vi "Hadamard vs DAQ (1).vi"() -> ()   [LabVIEW 2023]
uses:
  <vilib>/Utility/miscctls.llb/LVBoundsTypeDef.ctl
  <vilib>/Utility/miscctls.llb/LVRectTypeDef.ctl
panel:
  in  "Plot Area:Size":T1
  out "?":errorcluster
  in  "error in (no error)":errorcluster
  in  "Z Scale.Marker Values[]":cluster{dbl, u32}[](array[cluster])=[{0.0, 0}, {100.0, 16777215}]
  out "Delay":i32=20
  out "Intensity Graph":dbl[][](graph)=[[0.0, 1.0, 0.0, 1.0, 1.0, 0.0, 1.0, 0.0, 0.0, 1.0, 0.0, 1.0, 1.0, 0.0, 1.0, 0.0], [0.0, 1.0, 0.0, 1.0, 1.0, 0.0, 1.0, 0.0, 0.0, 1.0, 0.0, 1.0, 1.0, 0.0, 1.0, 0.0], [1.0, 0.0, 1.0, 0.0, 0.0, 1.0, 0.0, 1.0, 1.0, 0.0, 1.0, 0.0, 0.0, 1.0, 0.0, 1.0], [1.0, 0.0, 1.0, 0.0, 0.0, 1.0, 0.0, 1.0, 1.0, 0.0, 1.0, 0.0, 0.0, 1.0, 0.0, 1.0], [0.0, 1.0, 0.0, 1.0, 1.0, 0.0, 1.0, 0.0, 0.0, 1.0, 0.0, 1.0, 1.0, 0.0, 1.0, 0.0], [0.0, 1.0, 0.0, 1.0, 1.0, 0.0, 1.0, 0.0, 0.0, 1.0, 0.0, 1.0, 1.0, 0.0, 1.0, 0.0], [1.0, 0.0, 1.0, 0.0, 0.0, 1.0, 0.0, 1.0, 1.0, 0.0, 1.0, 0.0, 0.0, 1.0, 0.0, 1.0], [1.0, 0.0, 1.0, 0.0, 0.0, 1.0, 0.0, 1.0, 1.0, 0.0, 1.0, 0.0, 0.0, 1.0, 0.0, 1.0], [0.0, 1.0, 0.0, 1.0, 1.0, 0.0, 1.0, 0.0, 0.0, 1.0, 0.0, 1.0, 1.0, 0.0, 1.0, 0.0], [0.0, 1.0, 0.0, 1.0, 1.0, 0.0, 1.0, 0.0, 0.0, 1.0, 0.0, 1.0, 1.0, 0.0, 1.0, 0.0], [1.0, 0.0, 1.0, 0.0, 0.0, 1.0, 0.0, 1.0, 1.0, 0.0, 1.0, 0.0, 0.0, 1.0, 0.0, 1.0], [1.0, 0.0, 1.0, 0.0, 0.0, 1.0, 0.0, 1.0, 1.0, 0.0, 1.0, 0.0, 0.0, 1.0, 0.0, 1.0], [0.0, 1.0, 0.0, 1.0, 1.0, 0.0, 1.0, 0.0, 0.0, 1.0, 0.0, 1.0, 1.0, 0.0, 1.0, 0.0], [0.0, 1.0, 0.0, 1.0, 1.0, 0.0, 1.0, 0.0, 0.0, 1.0, 0.0, 1.0, 1.0, 0.0, 1.0, 0.0], [1.0, 0.0, 1.0, 0.0, 0.0, 1.0, 0.0, 1.0, 1.0, 0.0, 1.0, 0.0, 0.0, 1.0, 0.0, 1.0], [1.0, 0.0, 1.0, 0.0, 0.0, 1.0, 0.0, 1.0, 1.0, 0.0, 1.0, 0.0, 0.0, 1.0, 0.0, 1.0]]
  out "N":i32=16
  in  "stop":bool
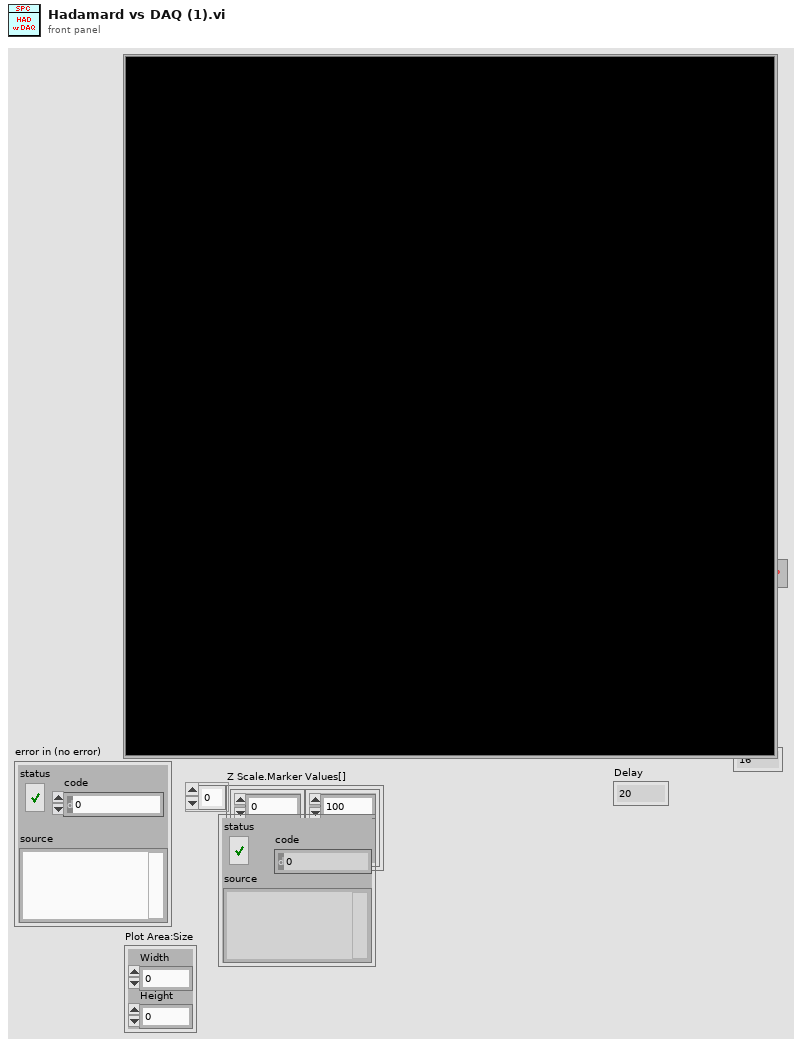
[diagram p1: front panel]
types:
  T1 = typedef "LVBoundsTypeDef.ctl" = cluster{"Width":u32, "Height":u32}
  T2 = typedef "LVRectTypeDef.ctl" = cluster{"Left":i16, "Top":i16, "Right":i16, "Bottom":i16}
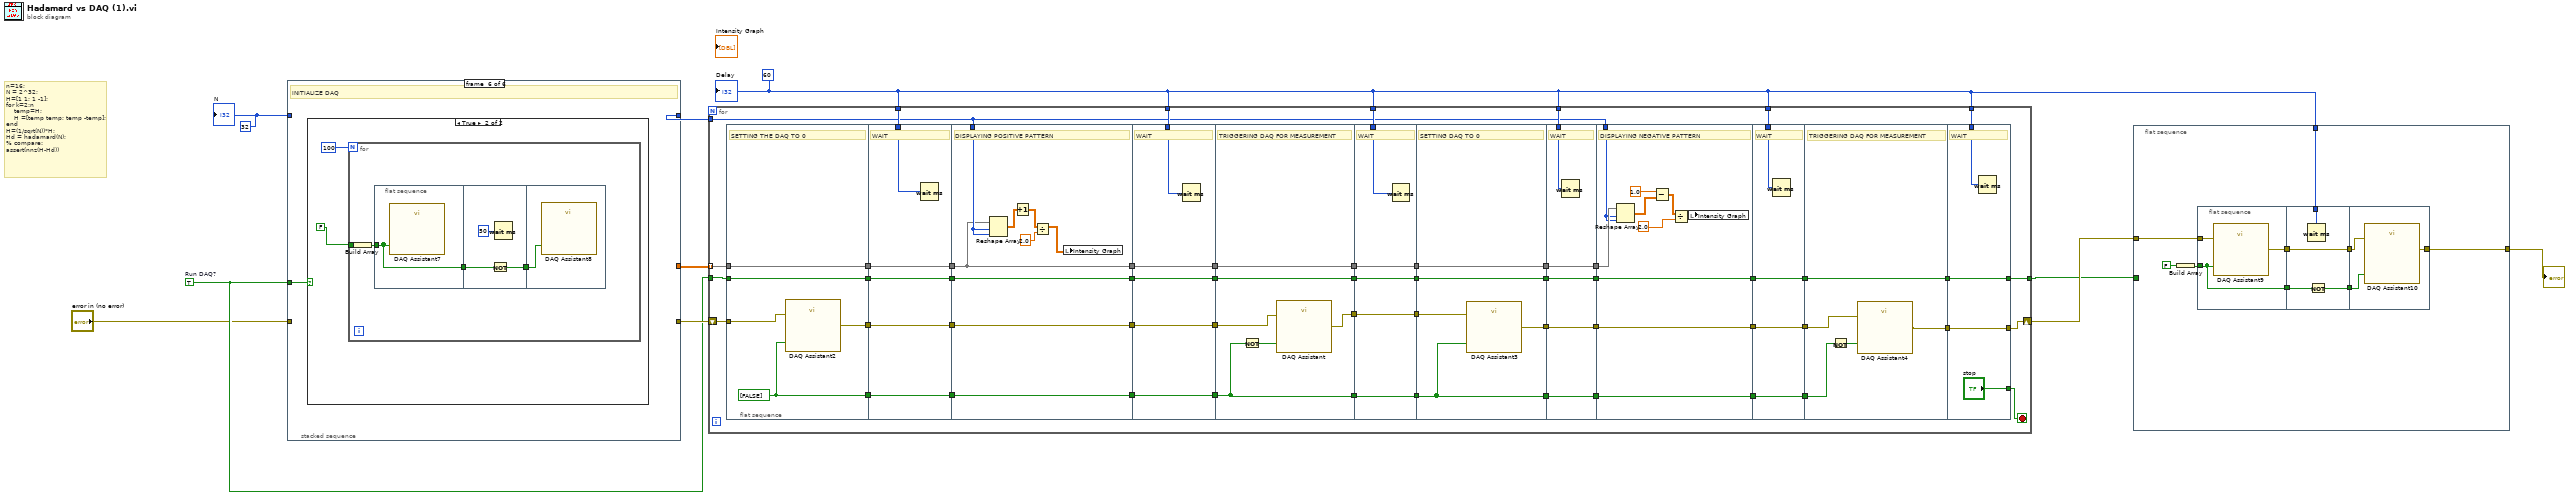
[diagram p0: block diagram]
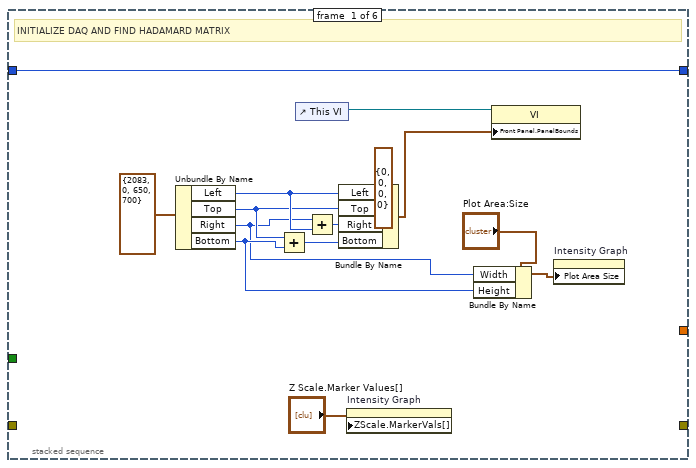
[diagram p2: hidden frame]
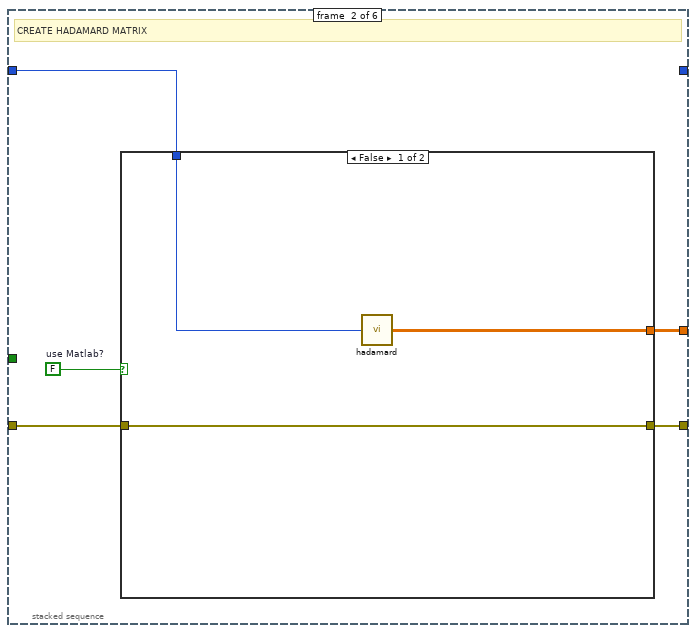
[diagram p3: hidden frame]
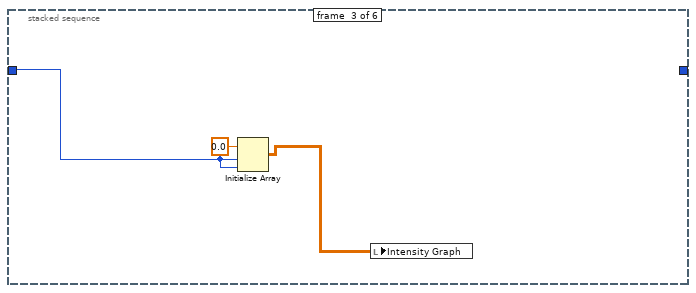
[diagram p5: hidden frame]
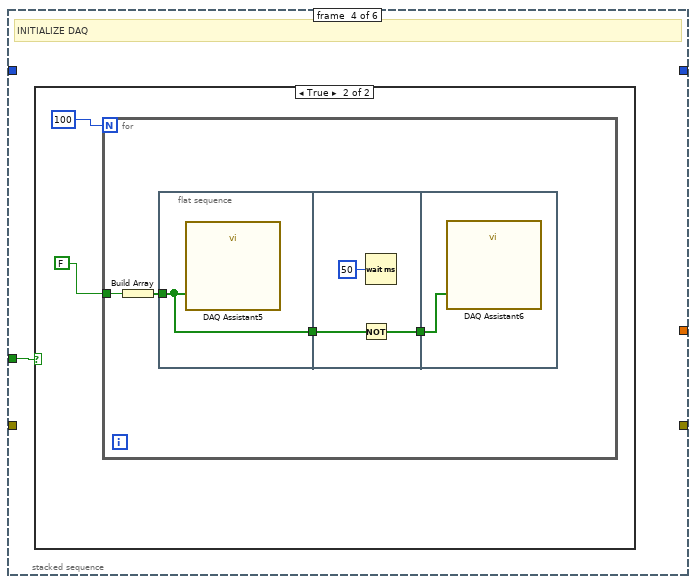
[diagram p6: hidden frame]
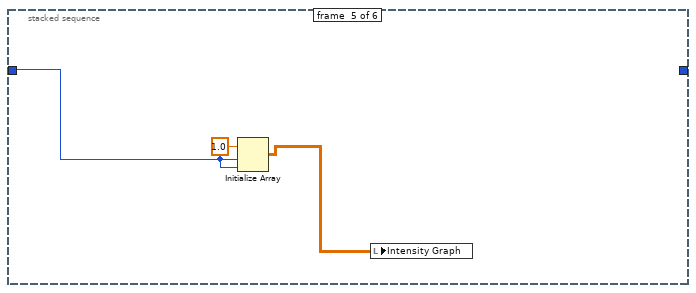
[diagram p8: hidden frame]
diagram:
  w4 = TRUE  # Run DAQ?
  w3 = 60 ("Delay")
  w7 = 32 ("N")
  # "n=16;\nN = 2^32;\nH=[1 1; 1 -1];\nfor k=2:n\n    temp=H;\n    H =[temp temp; temp -temp];\nend\nH=(1/sqrt(N))*H;\nHd = hadamard(N);\n% compare:\nassert(nnz(H-Hd))"
  n1 = stacked-sequence {
    tunnel: [_ w25 _ _ _ _] -> w9
    tunnel: w7 -> [w24 w28 w36 _ w51 _]
    tunnel: [w24 _ _ _ _ _] -> w8
    tunnel: [_ w27 _ _ _ _] -> w10
    tunnel: w4 -> [_ _ _ w37 _ w52]
    tunnel: "error in (no error)" -> [_ w26 _ _ _ _]
    frame #0 {
      # "INITIALIZE DAQ AND FIND HADAMARD MATRIX"
      n2 = Unbundle By Name(T2 {"Left"=2083, "Top"=0, "Right"=650, "Bottom"=700} ("Front Panel Window:Panel Bounds")) -> ("Left"=w20:i16, "Top"=w12:i16, "Right"=w11:i16, "Bottom"=w13:i16)
      n3 = Add(x=w12, y=w13) -> (x+y=w17:i16)
      n4 = control-ref of="This VI"() -> (w22:refnum<vi>)
      n5 = Add(x=w11, y=w20) -> (x+y=w19:i16)
      n6 = Bundle By Name(cluster=T2 {"Left"=0, "Top"=0, "Right"=0, "Bottom"=0} ("output cluster"), "Left"=w20, "Top"=w12, "Right"=w19, "Bottom"=w17) -> (w18:T2)
      n7 = property on="Intensity Graph" class="IntGraph (strict)"("ZScale.MarkerVals[]"="Z Scale.Marker Values[]") -> ()  [unwired: 2 in, 2 out]
      n8 = Bundle By Name(cluster="Plot Area:Size", "Width"=w11, "Height"=w13) -> (w14:T1)
      n9 = property class="VI"(reference=w22, "Front Panel.PanelBounds"=w18) -> ()  [unwired: 1 in, 2 out]
      n10 = property on="Intensity Graph" class="IntGraph (strict)"("Plot Area Size"=w14) -> ()  [unwired: 2 in, 2 out]
    }
    frame #1 {
      w29 = FALSE  # use Matlab?
      # "CREATE HADAMARD MATRIX"
      n11 = case shown="False" w29 {
        tunnel: w28 -> [w32 _]
        tunnel: [w31 _] -> w25
        tunnel: [w30 w33] -> w27
        tunnel: w26 -> [w30 w33]
        frame False {
          n12 = call "hadamard.vi"("N"=w32) -> ("Intensity Graph"=w31:dbl[][])
        }
        frame True {
          # "Copy this code to the matlab window"
        }
      }
    }
    frame #2 {
      n13 = Initialize Array(0.0 ("element"), w36, w36) -> (w35:dbl[][])
      n14 = local write "Intensity Graph"(w35) -> ()
    }
    frame #3 {
      # "INITIALIZE DAQ"
      n15 = case shown="True" w37 {
        frame False {
        }
        frame True {
          n16 = for {
            N: 100 -> [_]
            tunnel: FALSE -> [w42]
            n17 = Build Array(w42) -> (w43:bool[])
            n18 = flat-sequence {
              tunnel: w43 -> [w44]
              tunnel: [w44] -> w40
              tunnel: [w45] -> w41
              tunnel: w40 -> [w46]
              tunnel: w41 -> [w48]
              frame #0 {
                n19 = call "DAQ Assistant5"("data"=w44) -> ()  [unwired: 17 in, 2 out]
              }
              frame #1 {
                n20 = Not(x=w46) -> (.not. x?=w45:bool[])
                n21 = Wait (ms)(milliseconds to wait=u32 50) -> ()  [unwired: 1 out]
              }
              frame #2 {
                n22 = call "DAQ Assistant6"("data"=w48) -> ()  [unwired: 17 in, 2 out]
              }
            }
          }
        }
      }
    }
    frame #4 {
      n23 = Initialize Array(1.0 ("element"), w51, w51) -> (w50:dbl[][])
      n24 = local write "Intensity Graph"(w50) -> ()
    }
    frame #5 {
      # "INITIALIZE DAQ"
      n25 = case shown="True" w52 {
        frame False {
        }
        frame True {
          n26 = for {
            N: 100 -> [_]
            tunnel: FALSE -> [w57]
            n27 = Build Array(w57) -> (w58:bool[])
            n28 = flat-sequence {
              tunnel: w58 -> [w59]
              tunnel: [w59] -> w55
              tunnel: [w60] -> w56
              tunnel: w55 -> [w61]
              tunnel: w56 -> [w63]
              frame #0 {
                n29 = call "DAQ Assistant7"("data"=w59) -> ()  [unwired: 17 in, 2 out]
              }
              frame #1 {
                n30 = Not(x=w61) -> (.not. x?=w60:bool[])
                n31 = Wait (ms)(milliseconds to wait=u32 50) -> ()  [unwired: 1 out]
              }
              frame #2 {
                n32 = call "DAQ Assistant8"("data"=w63) -> ()  [unwired: 17 in, 2 out]
              }
            }
          }
        }
      }
    }
  }
  n33 = for {
    tunnel: w9 -> [w116] mode=indexing
    tunnel: w3 -> [w109]
    tunnel: w3 -> [w108]
    tunnel: w3 -> [w107]
    tunnel: w3 -> [w98]
    tunnel: w3 -> [w97]
    tunnel: w3 -> [w92]
    shift-right: [w90] -> w6
    shift-left: w10 -> [w78]
    tunnel: w8 -> [w77]
    tunnel: w4 -> [w76]
    tunnel: [w64] -> w2
    stop <- w91 stop-if-true
    n34 = flat-sequence {
      tunnel: w116 -> [w121]
      tunnel: [w121] -> w114
      tunnel: [w120] -> w110
      tunnel: [w119] -> w82
      tunnel: w78 -> [w118]
      tunnel: w76 -> [w117]
      tunnel: [w117] -> w72
      tunnel: [w126] -> w115
      tunnel: w114 -> [w126]
      tunnel: [w125] -> w111
      tunnel: w110 -> [w125]
      tunnel: w109 -> [w124]
      tunnel: w82 -> [w123]
      tunnel: [w123] -> w81
      tunnel: [w122] -> w73
      tunnel: w72 -> [w122]
      tunnel: w115 -> [w128]
      tunnel: w77 -> [w135]
      tunnel: [w134] -> w112
      tunnel: w111 -> [w134]
      tunnel: [w128] -> w104
      tunnel: w81 -> [w131]
      tunnel: [w131] -> w80
      tunnel: [w127] -> w74
      tunnel: w73 -> [w127]
      tunnel: [w140] -> w113
      tunnel: w112 -> [w140]
      tunnel: w108 -> [w139]
      tunnel: [w138] -> w105
      tunnel: w104 -> [w138]
      tunnel: w80 -> [w137]
      tunnel: [w137] -> w79
      tunnel: [w136] -> w75
      tunnel: w74 -> [w136]
      tunnel: w113 -> [w145]
      tunnel: [w146] -> w106
      tunnel: w105 -> [w146]
      tunnel: [w145] -> w101
      tunnel: [w144] -> w84
      tunnel: w79 -> [w143]
      tunnel: w75 -> [w142]
      tunnel: [w142] -> w70
      tunnel: w107 -> [w151]
      tunnel: [w150] -> w103
      tunnel: w106 -> [w150]
      tunnel: [w149] -> w102
      tunnel: w101 -> [w149]
      tunnel: w84 -> [w148]
      tunnel: [w148] -> w83
      tunnel: [w147] -> w71
      tunnel: w70 -> [w147]
      tunnel: w103 -> [w156]
      tunnel: [w156] -> w100
      tunnel: w102 -> [w155]
      tunnel: [w155] -> w93
      tunnel: [w154] -> w88
      tunnel: w83 -> [w153]
      tunnel: w71 -> [w152]
      tunnel: [w152] -> w65
      tunnel: w100 -> [w161]
      tunnel: [w161] -> w99
      tunnel: w98 -> [w160]
      tunnel: [w159] -> w94
      tunnel: w93 -> [w159]
      tunnel: w88 -> [w158]
      tunnel: [w158] -> w87
      tunnel: [w157] -> w66
      tunnel: w65 -> [w157]
      tunnel: w99 -> [w170]
      tunnel: w77 -> [w169]
      tunnel: [w167] -> w95
      tunnel: w94 -> [w167]
      tunnel: w87 -> [w166]
      tunnel: [w166] -> w86
      tunnel: [w162] -> w67
      tunnel: w66 -> [w162]
      tunnel: w97 -> [w175]
      tunnel: [w174] -> w96
      tunnel: w95 -> [w174]
      tunnel: w86 -> [w173]
      tunnel: [w173] -> w85
      tunnel: [w172] -> w68
      tunnel: w67 -> [w172]
      tunnel: w96 -> [w180]
      tunnel: [w179] -> w89
      tunnel: w85 -> [w176]
      tunnel: [w178] -> w69
      tunnel: w68 -> [w178]
      tunnel: w92 -> [w184]
      tunnel: ["stop"] -> w91
      tunnel: [w182] -> w90
      tunnel: w89 -> [w182]
      tunnel: [w181] -> w64
      tunnel: w69 -> [w181]
      frame #0 {
        w120 = bool[] [FALSE] ("data")
        # "SETTING THE DAQ TO 0"
        n35 = call "DAQ Assistant2"("data"=w120, "error in"=w118) -> ("error out"=w119:errorcluster)  [unwired: 16 in, 1 out]
      }
      frame #1 {
        # "WAIT"
        n36 = Wait (ms)(milliseconds to wait=w124) -> ()  [unwired: 1 out]
      }
      frame #2 {
        # "DISPLAYING POSITIVE PATTERN"
        n37 = Reshape Array(w128, w135, w135) -> (w130:dbl[][])
        n38 = Increment(x=w130) -> (x+1=w129:dbl[][])
        n39 = Divide(x=w129, y=2.0) -> (x/y=w132:dbl[][])
        n40 = local write "Intensity Graph"(w132) -> ()
      }
      frame #3 {
        # "WAIT"
        n41 = Wait (ms)(milliseconds to wait=w139) -> ()  [unwired: 1 out]
      }
      frame #4 {
        # "TRIGGERING DAQ FOR MEASUREMENT"
        n42 = Not(x=w145) -> (.not. x?=w141:bool[])
        n43 = call "DAQ Assistant"("data"=w141, "error in"=w143) -> ("error out"=w144:errorcluster)  [unwired: 16 in, 1 out]
      }
      frame #5 {
        # "WAIT"
        n44 = Wait (ms)(milliseconds to wait=w151) -> ()  [unwired: 1 out]
      }
      frame #6 {
        # "SETTING DAQ TO 0"
        n45 = call "DAQ Assistant3"("data"=w155, "error in"=w153) -> ("error out"=w154:errorcluster)  [unwired: 16 in, 1 out]
      }
      frame #7 {
        # "WAIT"
        n46 = Wait (ms)(milliseconds to wait=w160) -> ()  [unwired: 1 out]
      }
      frame #8 {
        # "DISPLAYING NEGATIVE PATTERN"
        n47 = Reshape Array(w170, w169, w169) -> (w164:dbl[][])
        n48 = Subtract(x=1.0, y=w164) -> (x-y=w163:dbl[][])
        n49 = Divide(x=w163, y=2.0) -> (x/y=w168:dbl[][])
        n50 = local write "Intensity Graph"(w168) -> ()
      }
      frame #9 {
        # "WAIT"
        n51 = Wait (ms)(milliseconds to wait=w175) -> ()  [unwired: 1 out]
      }
      frame #10 {
        # "TRIGGERING DAQ FOR MEASUREMENT"
        n52 = Not(x=w180) -> (.not. x?=w177:bool[])
        n53 = call "DAQ Assistant4"("data"=w177, "error in"=w176) -> ("error out"=w179:errorcluster)  [unwired: 16 in, 1 out]
      }
      frame #11 {
        # "WAIT"
        n54 = Wait (ms)(milliseconds to wait=w184) -> ()  [unwired: 1 out]
      }
    }
  }
  n55 = flat-sequence {
    tunnel: w6 -> [w193]
    tunnel: [w192] -> w5
    tunnel: w3 -> [w191]
    tunnel: w2 -> [_]
    frame #0 {
      n56 = Build Array(FALSE) -> (w185:bool[])
      n57 = flat-sequence {
        tunnel: w185 -> [w196]
        tunnel: [w196] -> w190
        tunnel: w193 -> [w195]
        tunnel: [w194] -> w189
        tunnel: [w199] -> w188
        tunnel: w190 -> [w200]
        tunnel: [w198] -> w187
        tunnel: w189 -> [w198]
        tunnel: w191 -> [w197]
        tunnel: w188 -> [w203]
        tunnel: w187 -> [w202]
        tunnel: [w201] -> w192
        frame #0 {
          n58 = call "DAQ Assistant9"("data"=w196, "error in"=w195) -> ("error out"=w194:errorcluster)  [unwired: 16 in, 1 out]
        }
        frame #1 {
          n59 = Wait (ms)(milliseconds to wait=w197) -> ()  [unwired: 1 out]
          n60 = Not(x=w200) -> (.not. x?=w199:bool[])
        }
        frame #2 {
          n61 = call "DAQ Assistant10"("data"=w203, "error in"=w202) -> ("error out"=w201:errorcluster)  [unwired: 16 in, 1 out]
        }
      }
    }
  }
  "N" <- w7
  "Delay" <- w3
  "?" <- w5
